vi "zadanie 1.vi"() -> ()   [LabVIEW 2013]
panel:
  out "initialized array":dbl[](array[numeric])
  in  "Numeric":dbl
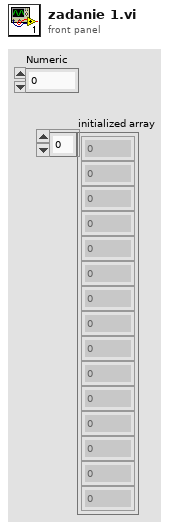
[diagram p1: front panel]
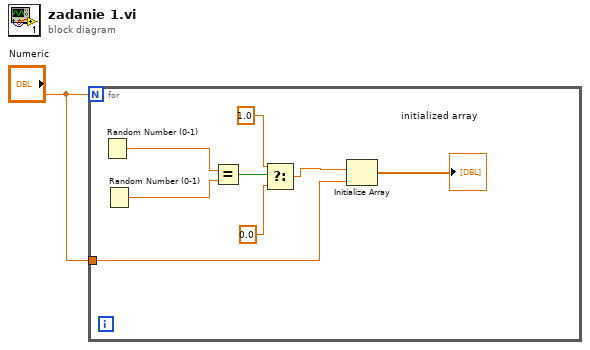
[diagram p0: block diagram]
diagram:
  n1 = for {
    N: "Numeric" -> [_]
    tunnel: "Numeric" -> [w2]
    n2 = Random Number (0-1)() -> (number: 0 to 1=w9:dbl)
    n3 = Random Number (0-1)() -> (number: 0 to 1=w8:dbl)
    n4 = Equal?(x=w9, y=w8) -> (x = y?=w5:bool)
    n5 = Select(t=1.0, s=w5, f=0.0) -> (s? t:f=w4:dbl)
    n6 = Initialize Array(w4, w2) -> (→"initialized array":dbl[])
  }
